vi "ParseSwerveModuleCurrentLimit.vi"(8 "moduleName":string, 9 "configRef":T1) -> (2 "outputCluster":T2, 3 "configRefOut":T1)   [LabVIEW 2020]
uses:
  <vilib>/Utility/config.llb/Config Data RefNum.ctl
  <vilib>/Rock Robotics/WPI/ThirdParty/Phoenix-LabVIEW/Motor Controller/Controls/CTRE_Phoenix_MotorControl_SupplyCurrentLimitConfiguration.ctl
  <vilib>/Utility/config.llb/Read Key (Double).vi
  <vilib>/Utility/config.llb/Read Key (Boolean).vi
  <vilib>/Utility/config.llb/NI_LVConfig.lvlib
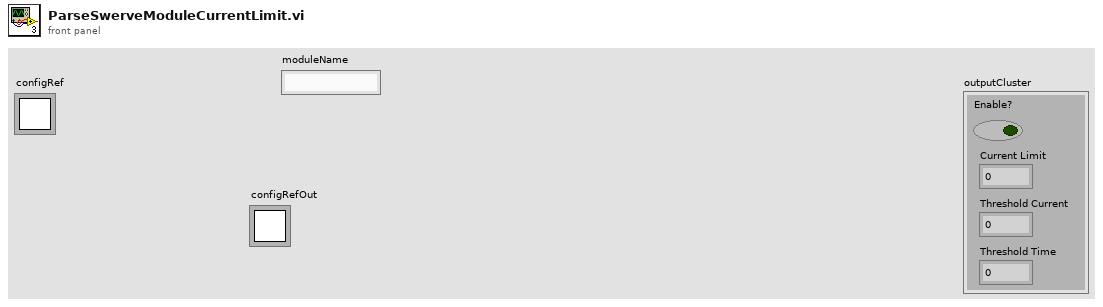
[diagram p1: front panel]
types:
  T1 = typedef "NI_LVConfig.lvlib/Config Data RefNum.ctl" = refnum<k1>
  T2 = typedef "CTRE_Phoenix_MotorControl_SupplyCurrentLimitConfiguration.ctl" = cluster{"Enable?":bool, "Current Limit":dbl, "Threshold Current":dbl, "Threshold Time":dbl}
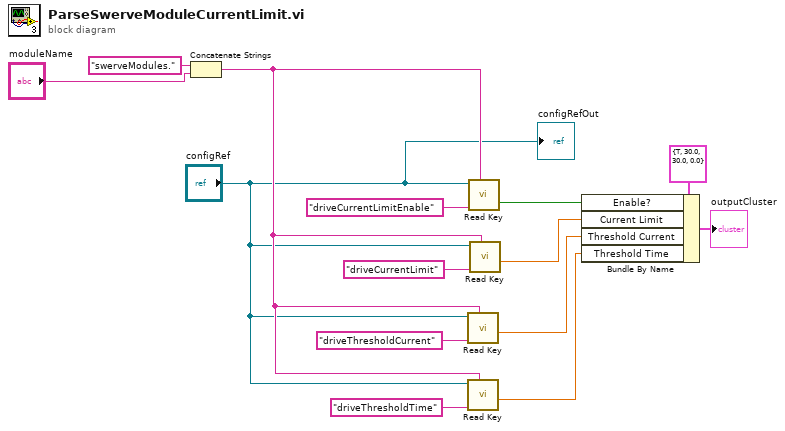
[diagram p0: block diagram]
diagram:
  n1 = Concatenate Strings("swerveModules." ("string"), "moduleName") -> (w3:string)
  n2 = call-poly <vilib>:"Read Key.vi"("section"=w3, "key"="driveThresholdCurrent", "refnum"="configRef") -> ("value"=w5:dbl)  [unwired: 5 in, 3 out]
  n3 = call-poly <vilib>:"Read Key.vi"("section"=w3, "key"="driveThresholdTime", "refnum"="configRef") -> ("value"=w2:dbl)  [unwired: 5 in, 3 out]
  n4 = call-poly <vilib>:"Read Key.vi"("section"=w3, "key"="driveCurrentLimitEnable", "refnum"="configRef") -> ("value"=w10:bool)  [unwired: 5 in, 3 out]
  n5 = call-poly <vilib>:"Read Key.vi"("section"=w3, "key"="driveCurrentLimit", "refnum"="configRef") -> ("value"=w7:dbl)  [unwired: 5 in, 3 out]
  n6 = Bundle By Name(cluster=T2 {"Enable?"=TRUE, "Current Limit"=30.0, "Threshold Current"=30.0, "Threshold Time"=0.0} ("driveCurrentLimitConfig"), "Enable?"=w10, "Current Limit"=w7, "Threshold Current"=w5, "Threshold Time"=w2) -> (→"outputCluster":T2)
  "configRefOut" <- "configRef"
